vi "tdmsGenToolScaleAllDAQmxTypes.vi"() -> ()   [LabVIEW 2026]
uses:
  <vilib>/Platform/TimedLoop/XDataNode/nitl_modes.ctl
  <vilib>/Platform/TimedLoop/XDataNode/timing_clust.ctl
  <vilib>/Platform/TimedLoop/XDataNode/wakeup.ctl
  <vilib>/DAQmx/read.llb/DAQmx Read (Analog 1D DBL 1Chan NSamp).vi
  <vilib>/DAQmx/create/scale.llb/DAQmx Create Scale (Map Ranges).vi
  <vilib>/DAQmx/create/channels.llb/DAQmx Create Channel (AI-Voltage-Basic).vi
  <vilib>/DAQmx/create/channels.llb/DAQmx Create Channel (AI-Strain-Strain Gage).vi
  <vilib>/DAQmx/create/channels.llb/DAQmx Create Channel (AI-Current-Basic).vi
  <vilib>/DAQmx/create/channels.llb/DAQmx Create Channel (AI-Temperature-RTD).vi
  <vilib>/DAQmx/create/channels.llb/DAQmx Create Channel (AI-Temperature-Thermocouple).vi
  <vilib>/DAQmx/configure/timing.llb/DAQmx Timing (Sample Clock).vi
  <vilib>/DAQmx/configure/task.llb/DAQmx Configure Logging (TDMS).vi
  <vilib>/DAQmx/miscellaneous.llb/DAQmx Fill In Error Info.vi
  <vilib>/platform/TimedLoop/XDataNode/XDataNode.xnode
  <vilib>/Platform/TimedLoop/XDataNode/XDNodeRunTimeDep.lvlib
  <resource>/objmgr/daqmx.rc
panel:
  out "Numeric":i32
  out "Waveform Chart":dbl[](graph)
  in  "DAQType Enum":T1(ring)
  in  "double?":bool
  in  "file format version (2.0)":enum16{"1.0", "2.0"}(ring)=enum."2.0"
  in  "create index file? (T)":bool=TRUE
  in  "byte order (2:little-endian)":T2(ring)
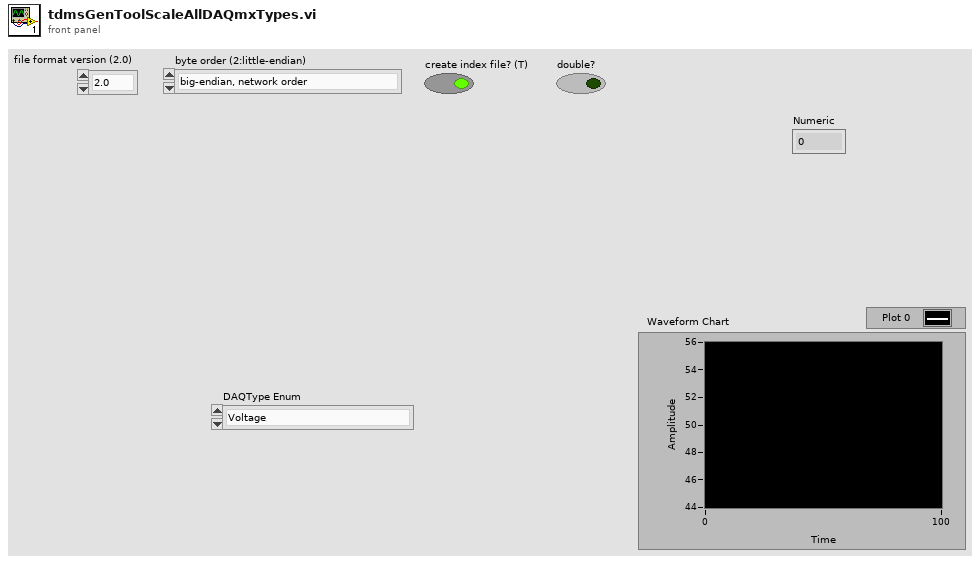
[diagram p1: front panel]
types:
  T1 = enum16{"Voltage", "Current", "RTD", "Thermocouple", "Strain"}
  T2 = enum16{"big-endian, network order", "native, host order", "little-endian"}
  T3 = cluster{"gage factor":dbl, "nominal gage resistance":dbl, "poisson ratio":dbl}
  T4 = typedef "XDNodeRunTimeDep.lvlib/nitl_modes.ctl" = enum32{"No Change", "Process missed periods, maintain original phase", "Discard missed periods, maintain original phase", "Process missed periods, ignore original phase", "Discard missed periods, ignore original phase"}
  T5 = typedef "XDNodeRunTimeDep.lvlib/timing_clust.ctl" = cluster{"Expected End [f-1]":u64, "Actual End [f-1]":u64, "Finished Late? [f-1]":bool, "Expected End [i-1]":u64, "Actual End [i-1]":u64, "Finished Late? [i-1]":bool, "Expected Start [i]":u64, "Actual Start [i]":u64, "Expected Start [f]":u64, "Actual Start [f]":u64, "Source Name":string, "Structure Name":string, "Period":i64, "Deadline":i64, "Offset":i64, "Start":i64, "Priority":i32, "Timeout":i32, "Mode":T4, "Wakeup Reason":T6, "Error":errorcluster, "Source Type":string, "Secondary Source Type":string, "Global End Time":u64, "Global Start Time":u64, "Frame Duration":u64, "Iteration Duration":u64, "Assigned CPU":i32, "I/O Scan Engine Mode":u32}
  T6 = typedef "XDNodeRunTimeDep.lvlib/wakeup.ctl" = enum32{"Normal", "Aborted", "Asynchronous wakeup", "Timing source error", "Timed loop error", "Timeout"}
  T7 = enum16{"open", "open or create", "create or replace", "create", "open (read-only)"}
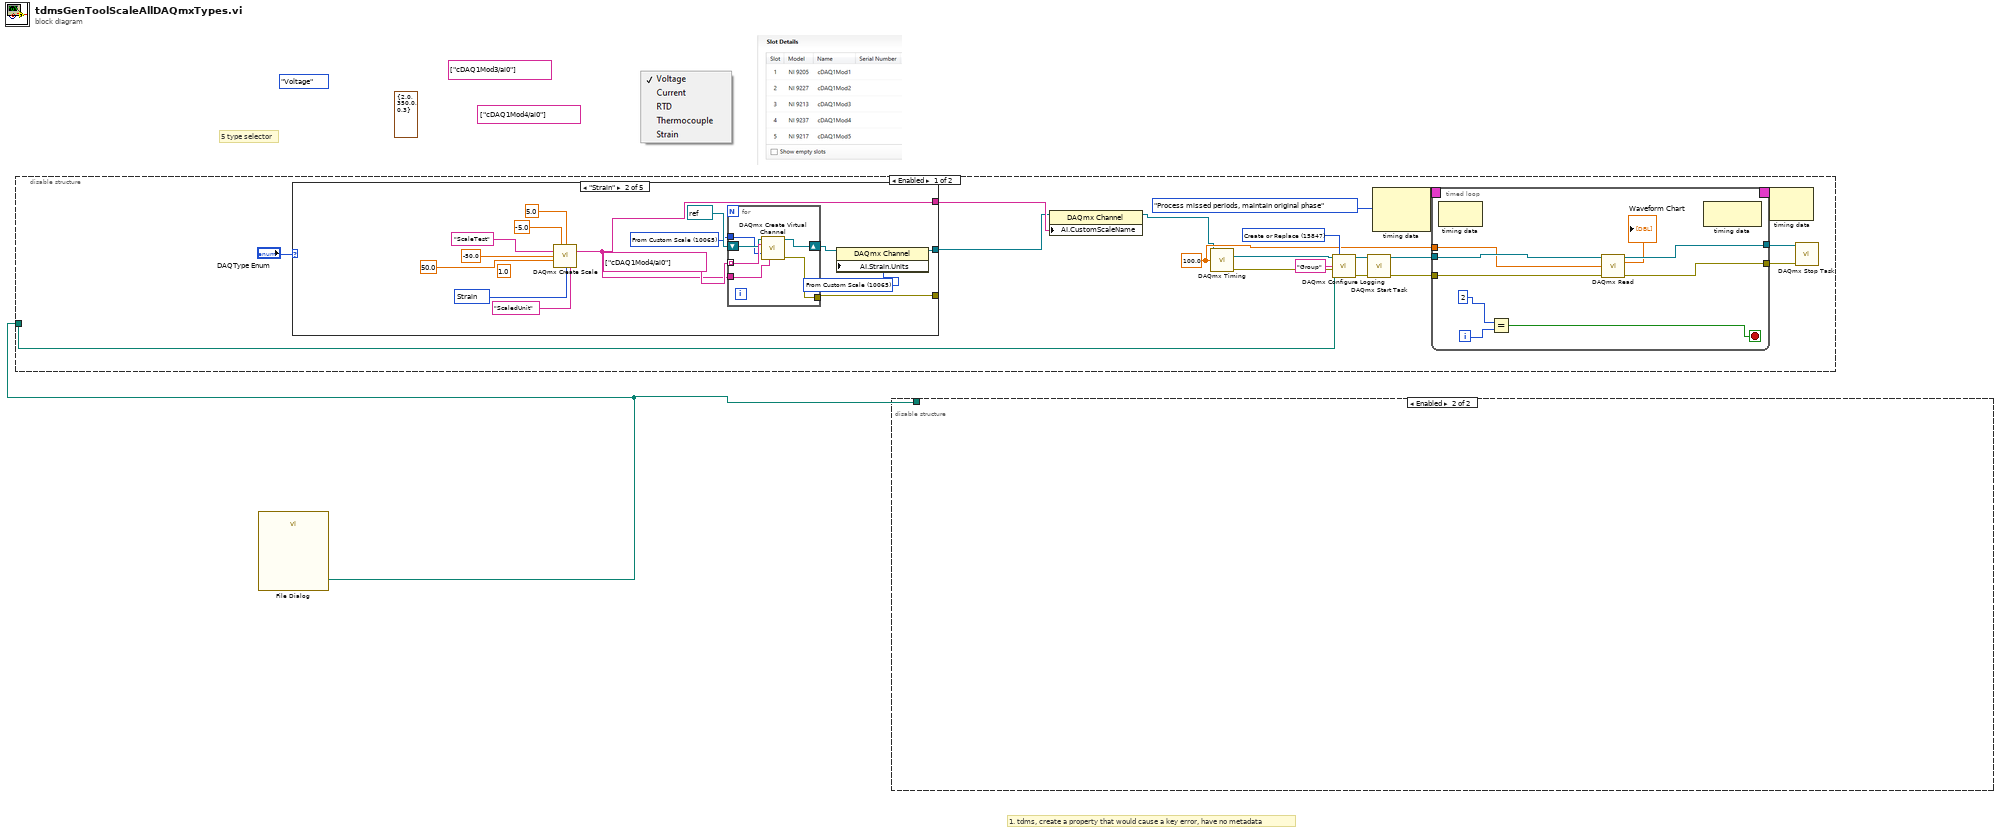
[diagram p0: block diagram]
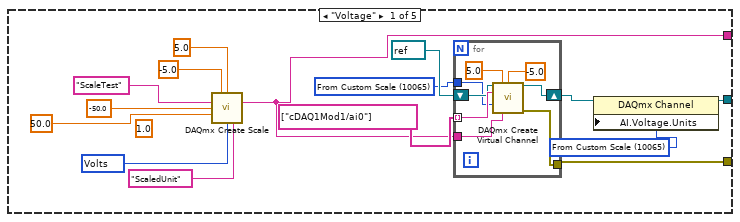
[diagram p2: hidden frame]
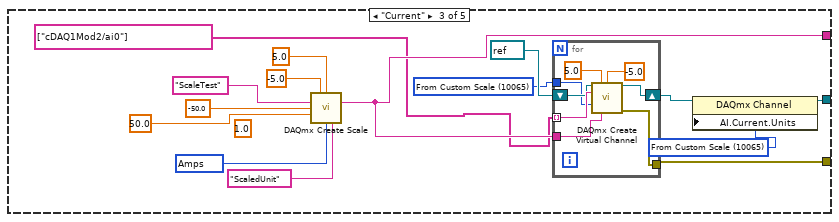
[diagram p3: hidden frame]
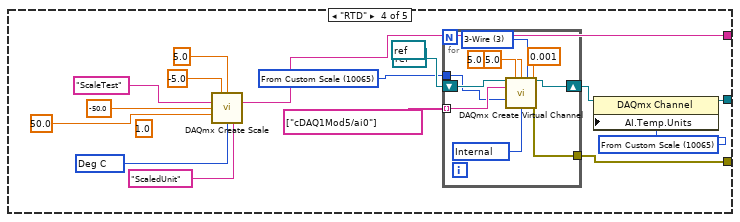
[diagram p4: hidden frame]
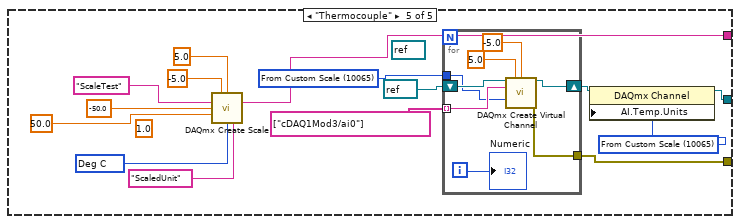
[diagram p5: hidden frame]
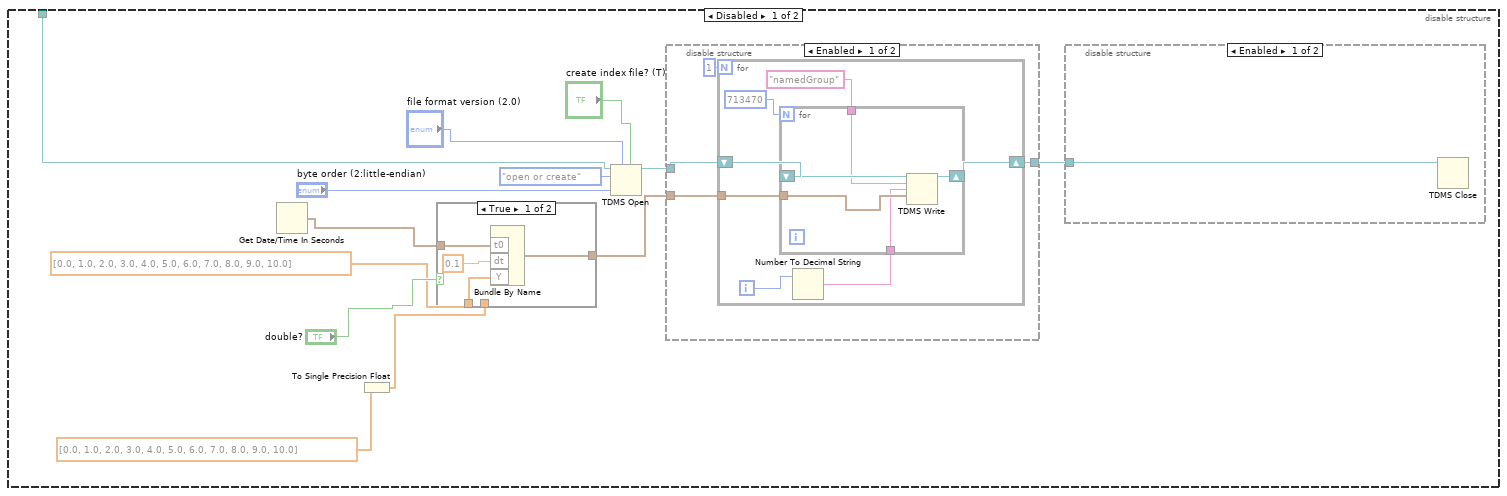
[diagram p7: hidden frame]
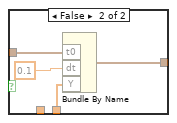
[diagram p10: hidden frame]
diagram:
  (unwired) tag[] ["cDAQ1Mod4/ai0"] ("Voltage Channels")
  (unwired) T3 {"gage factor"=2.0, "nominal gage resistance"=350.0, "poisson ratio"=0.3} ("strain gage information")
  (unwired) tag[] ["cDAQ1Mod3/ai0"] ("Voltage Channels")
  (unwired) T1."Voltage"
  # "5 type selector"
  # "1. tdms, create a property that would cause a key error, have no metadata"
  n1 = call "File Dialog"() -> ("selected path"=w1:path)  [unwired: 12 in, 3 out]
  n2 = disable-structure shown="Enabled" {
    disable-tunnel: w1 -> [w6 _]
    frame Enabled {
      w18 = 15847 items=["Open"=10437, "Open or Create"=15846, "Create or Replace"=15847, "Create"=15848] ("operation")
      w5 = 100.0 ("rate")
      n3 = case shown="\"Strain\"" "DAQType Enum" {
        tunnel: [w30 w53 w75 w102 w127] -> w2
        tunnel: [w35 w58 w79 w88 w113] -> _
        tunnel: [w25 w48 w70 w97 w122] -> w3
        frame "Voltage" {
          (unwired) 1.0 ("y-intercept")
          w29 = 10065 items=["Volts"=10348, "From Custom Scale"=10065, "From TEDS"=12516] ("AI.Voltage.Units")
          w26 = 10348 items=["Volts"=10348, "Amps"=10342, "Watts"=16203, "Deg F"=10144, "Deg C"=10143, "Deg R"=10145, "Kelvins"=10325, "Strain"=10299, "Ohms"=10384, "Hz"=10373, "Seconds"=10364, "Meters"=10219, "Inches"=10379, "Degrees"=10146, "Radians"=10273, "Ticks"=10304, "g"=10186, "m/s^2"=12470, "m/s"=15959, "in/s"=15960, "Pascals"=10081, "Newtons"=15875, "Pounds"=15876, "kgf"=15877, "psi"=15879, "bar"=15880, "Nm"=15881, "oz-in"=15882, "lb-in"=15883, "lb-ft"=15884, "Volts/Volt"=15896, "mVolts/Volt"=15897, "pCoulombs"=16103, "Coulombs"=16102, "From TEDS"=12516] ("pre-scaled units")
          w32 = 10065 items=["Volts"=10348, "From Custom Scale"=10065] ("units")
          n4 = call-poly <vilib>:"DAQmx Create Scale.vi"("pre-scaled minimum"=-5.0, "pre-scaled maximum"=5.0, "name"="ScaleTest", "scaled minimum"=-50.0, "scaled maximum"=50.0, "pre-scaled units"=w26, "scaled units"="ScaledUnit") -> ("scale out"=w25:tag)  [unwired: 7 in, 1 out]
          n5 = for {
            tunnel: [w42] -> w35
            tunnel: tag[] ["cDAQ1Mod1/ai0"] ("Voltage Channels") -> [w41] mode=indexing
            shift-right: [w43] -> w31
            shift-left: refnum<k21> refnum ("task out") -> [w40]
            tunnel: w32 -> [w39]
            tunnel: w25 -> [w38]
            n6 = call-poly <vilib>:"DAQmx Create Virtual Channel.vi"("task in"=w40, "maximum value"=5.0, "minimum value"=-5.0, "physical channels"=w41, "units"=w39, "custom scale name"=w38) -> ("task out"=w43:refnum<k21>, "error out"=w42:errorcluster)  [unwired: 8 in]
          }
          n7 = property class="DAQmx Channel"(reference=w31, "AI.Voltage.Units"=w29) -> (reference out=w30:refnum<k21>)  [unwired: 1 in, 1 out]
        }
        frame "Strain" {
          (unwired) 1.0 ("y-intercept")
          w52 = 10065 items=["Volts"=10348, "From Custom Scale"=10065, "From TEDS"=12516] ("AI.Voltage.Units")
          w49 = 10299 items=["Volts"=10348, "Amps"=10342, "Watts"=16203, "Deg F"=10144, "Deg C"=10143, "Deg R"=10145, "Kelvins"=10325, "Strain"=10299, "Ohms"=10384, "Hz"=10373, "Seconds"=10364, "Meters"=10219, "Inches"=10379, "Degrees"=10146, "Radians"=10273, "Ticks"=10304, "g"=10186, "m/s^2"=12470, "m/s"=15959, "in/s"=15960, "Pascals"=10081, "Newtons"=15875, "Pounds"=15876, "kgf"=15877, "psi"=15879, "bar"=15880, "Nm"=15881, "oz-in"=15882, "lb-in"=15883, "lb-ft"=15884, "Volts/Volt"=15896, "mVolts/Volt"=15897, "pCoulombs"=16103, "Coulombs"=16102, "From TEDS"=12516] ("pre-scaled units")
          w55 = 10065 items=["Volts"=10348, "From Custom Scale"=10065] ("units")
          n8 = call-poly <vilib>:"DAQmx Create Scale.vi"("pre-scaled minimum"=-5.0, "pre-scaled maximum"=5.0, "name"="ScaleTest", "scaled minimum"=-50.0, "scaled maximum"=50.0, "pre-scaled units"=w49, "scaled units"="ScaledUnit") -> ("scale out"=w48:tag)  [unwired: 7 in, 1 out]
          n9 = for {
            tunnel: [w63] -> w58
            tunnel: tag[] ["cDAQ1Mod4/ai0"] ("Voltage Channels") -> [w62] mode=indexing
            shift-right: [w64] -> w54
            shift-left: refnum<k21> refnum ("task out") -> [w61]
            tunnel: w55 -> [w60]
            tunnel: w48 -> [w59]
            n10 = call-poly <vilib>:"DAQmx Create Virtual Channel.vi"("task in"=w61, "physical channels"=w62, "units"=w60, "custom scale name"=w59) -> ("task out"=w64:refnum<k21>, "error out"=w63:errorcluster)  [unwired: 10 in]
          }
          n11 = property class="DAQmx Channel"(reference=w54, "AI.Strain.Units"=w52) -> (reference out=w53:refnum<k21>)  [unwired: 1 in, 1 out]
        }
        frame "Current" {
          (unwired) 1.0 ("y-intercept")
          w74 = 10065 items=["Volts"=10348, "From Custom Scale"=10065, "From TEDS"=12516] ("AI.Voltage.Units")
          w71 = 10342 items=["Volts"=10348, "Amps"=10342, "Watts"=16203, "Deg F"=10144, "Deg C"=10143, "Deg R"=10145, "Kelvins"=10325, "Strain"=10299, "Ohms"=10384, "Hz"=10373, "Seconds"=10364, "Meters"=10219, "Inches"=10379, "Degrees"=10146, "Radians"=10273, "Ticks"=10304, "g"=10186, "m/s^2"=12470, "m/s"=15959, "in/s"=15960, "Pascals"=10081, "Newtons"=15875, "Pounds"=15876, "kgf"=15877, "psi"=15879, "bar"=15880, "Nm"=15881, "oz-in"=15882, "lb-in"=15883, "lb-ft"=15884, "Volts/Volt"=15896, "mVolts/Volt"=15897, "pCoulombs"=16103, "Coulombs"=16102, "From TEDS"=12516] ("pre-scaled units")
          w77 = 10065 items=["Volts"=10348, "From Custom Scale"=10065] ("units")
          n12 = call-poly <vilib>:"DAQmx Create Scale.vi"("pre-scaled minimum"=-5.0, "pre-scaled maximum"=5.0, "name"="ScaleTest", "scaled minimum"=-50.0, "scaled maximum"=50.0, "pre-scaled units"=w71, "scaled units"="ScaledUnit") -> ("scale out"=w70:tag)  [unwired: 7 in, 1 out]
          n13 = for {
            tunnel: [w86] -> w79
            tunnel: tag[] ["cDAQ1Mod2/ai0"] ("Voltage Channels") -> [w85] mode=indexing
            shift-right: [w87] -> w76
            shift-left: refnum<k21> refnum ("task out") -> [w84]
            tunnel: w77 -> [w83]
            tunnel: w70 -> [w82]
            n14 = call-poly <vilib>:"DAQmx Create Virtual Channel.vi"("task in"=w84, "maximum value"=5.0, "minimum value"=-5.0, "physical channels"=w85, "units"=w83, "custom scale name"=w82) -> ("task out"=w87:refnum<k21>, "error out"=w86:errorcluster)  [unwired: 8 in]
          }
          n15 = property class="DAQmx Channel"(reference=w76, "AI.Current.Units"=w74) -> (reference out=w75:refnum<k21>)  [unwired: 1 in, 1 out]
        }
        frame "RTD" {
          (unwired) 1.0 ("y-intercept")
          w101 = 10065 items=["Volts"=10348, "From Custom Scale"=10065, "From TEDS"=12516] ("AI.Voltage.Units")
          w98 = 10143 items=["Volts"=10348, "Amps"=10342, "Watts"=16203, "Deg F"=10144, "Deg C"=10143, "Deg R"=10145, "Kelvins"=10325, "Strain"=10299, "Ohms"=10384, "Hz"=10373, "Seconds"=10364, "Meters"=10219, "Inches"=10379, "Degrees"=10146, "Radians"=10273, "Ticks"=10304, "g"=10186, "m/s^2"=12470, "m/s"=15959, "in/s"=15960, "Pascals"=10081, "Newtons"=15875, "Pounds"=15876, "kgf"=15877, "psi"=15879, "bar"=15880, "Nm"=15881, "oz-in"=15882, "lb-in"=15883, "lb-ft"=15884, "Volts/Volt"=15896, "mVolts/Volt"=15897, "pCoulombs"=16103, "Coulombs"=16102, "From TEDS"=12516] ("pre-scaled units")
          w90 = 10065 items=["Volts"=10348, "From Custom Scale"=10065] ("units")
          (unwired) refnum<k21> refnum ("task out")
          n16 = call-poly <vilib>:"DAQmx Create Scale.vi"("pre-scaled minimum"=-5.0, "pre-scaled maximum"=5.0, "name"="ScaleTest", "scaled minimum"=-50.0, "scaled maximum"=50.0, "pre-scaled units"=w98, "scaled units"="ScaledUnit") -> ("scale out"=w97:tag)  [unwired: 7 in, 1 out]
          n17 = for {
            tunnel: [w111] -> w88
            tunnel: tag[] ["cDAQ1Mod5/ai0"] ("Voltage Channels") -> [w110] mode=indexing
            shift-right: [w112] -> w89
            shift-left: refnum<k21> refnum ("task out") -> [w109]
            tunnel: w90 -> [w105]
            w106 = 3 items=["2-Wire"=2, "3-Wire"=3, "4-Wire"=4] ("resistance configuration")
            w108 = 10200 items=["Internal"=10200, "External"=10167, "None"=10230] ("current excitation source")
            n18 = call-poly <vilib>:"DAQmx Create Virtual Channel.vi"("task in"=w109, "maximum value"=5.0, "minimum value"=-5.0, "resistance configuration"=w106, "physical channels"=w110, "units"=w105, "current excitation value"=0.001, "current excitation source"=w108) -> ("task out"=w112:refnum<k21>, "error out"=w111:errorcluster)  [unwired: 6 in]
          }
          n19 = property class="DAQmx Channel"(reference=w89, "AI.Temp.Units"=w101) -> (reference out=w102:refnum<k21>)  [unwired: 1 in, 1 out]
        }
        frame "Thermocouple" {
          (unwired) 1.0 ("y-intercept")
          w126 = 10065 items=["Volts"=10348, "From Custom Scale"=10065, "From TEDS"=12516] ("AI.Voltage.Units")
          w123 = 10143 items=["Volts"=10348, "Amps"=10342, "Watts"=16203, "Deg F"=10144, "Deg C"=10143, "Deg R"=10145, "Kelvins"=10325, "Strain"=10299, "Ohms"=10384, "Hz"=10373, "Seconds"=10364, "Meters"=10219, "Inches"=10379, "Degrees"=10146, "Radians"=10273, "Ticks"=10304, "g"=10186, "m/s^2"=12470, "m/s"=15959, "in/s"=15960, "Pascals"=10081, "Newtons"=15875, "Pounds"=15876, "kgf"=15877, "psi"=15879, "bar"=15880, "Nm"=15881, "oz-in"=15882, "lb-in"=15883, "lb-ft"=15884, "Volts/Volt"=15896, "mVolts/Volt"=15897, "pCoulombs"=16103, "Coulombs"=16102, "From TEDS"=12516] ("pre-scaled units")
          w115 = 10065 items=["Volts"=10348, "From Custom Scale"=10065] ("units")
          (unwired) refnum<k21> refnum ("task out")
          n20 = call-poly <vilib>:"DAQmx Create Scale.vi"("pre-scaled minimum"=-5.0, "pre-scaled maximum"=5.0, "name"="ScaleTest", "scaled minimum"=-50.0, "scaled maximum"=50.0, "pre-scaled units"=w123, "scaled units"="ScaledUnit") -> ("scale out"=w122:tag)  [unwired: 7 in, 1 out]
          n21 = for {
            tunnel: [w134] -> w113
            tunnel: tag[] ["cDAQ1Mod3/ai0"] ("Voltage Channels") -> [w133] mode=indexing
            shift-right: [w135] -> w114
            shift-left: refnum<k21> refnum ("task out") -> [w132]
            tunnel: w115 -> [w131]
            i -> [w128]
            n22 = call-poly <vilib>:"DAQmx Create Virtual Channel.vi"("task in"=w132, "maximum value"=5.0, "minimum value"=-5.0, "physical channels"=w133, "units"=w131) -> ("task out"=w135:refnum<k21>, "error out"=w134:errorcluster)  [unwired: 9 in]
            "Numeric" <- w128
          }
          n23 = property class="DAQmx Channel"(reference=w114, "AI.Temp.Units"=w126) -> (reference out=w127:refnum<k21>)  [unwired: 1 in, 1 out]
        }
      }
      n24 = property class="DAQmx Channel"(reference=w2, "AI.CustomScaleName"=w3) -> (reference out=w4:refnum<k21>)  [unwired: 1 in, 1 out]
      n25 = call-poly <vilib>:"DAQmx Timing.vi"("task/channels in"=w4, "rate"=w5) -> ("task out"=w16:refnum<k21>, "error out"=w15:errorcluster)  [unwired: 12 in]
      n26 = call-poly <vilib>:"DAQmx Configure Logging.vi"("task/channels in"=w16, "operation"=w18, "file path"=w6, "group name"="Group", "error in"=w15) -> ("task out"=w14:refnum<k21>, "error out"=w13:errorcluster)  [unwired: 9 in]
      n27 = call <vilib>:"DAQmx Start Task.vi"("task/channels in"=w14, "error in"=w13) -> ("task out"=w12:refnum<k21>, "error out"=w11:errorcluster)  [unwired: 12 in]
      n28 = node-c288(nitl_modes."Process missed periods, maintain original phase" ("Mode")) -> (w20:T5)  [unwired: 1 in]
      n29 = timed-loop {
        tunnel: w12 -> [w141]
        tunnel: w11 -> [w140]
        timing: w20 -> [_]
        timing-out: [_] -> w19
        tunnel: [w139] -> w10
        tunnel: [w138] -> w9
        tunnel: w5 -> [w137]
        i -> [w144]
        stop <- w143 stop-if-true
        n30 = node-c288() -> ()  [unwired: 1 in, 1 out]
        n31 = Equal?(x=2, y=w144) -> (x = y?=w143:bool)
        n32 = call-poly <vilib>:"DAQmx Read.vi"("task/channels in"=w141, "number of samples per channel"=w137, "error in"=w140) -> ("task out"=w139:refnum<k21>, "data"=→"Waveform Chart":dbl[], "error out"=w138:errorcluster)  [unwired: 10 in]
        n33 = node-c288() -> ()  [unwired: 1 in, 1 out]
      }
      n34 = node-c288(w19) -> ()  [unwired: 1 out]
      n35 = call <vilib>:"DAQmx Stop Task.vi"("task/channels in"=w10, "error in"=w9) -> ()  [unwired: 12 in, 2 out]
    }
    frame Disabled {
    }
  }
  n36 = disable-structure shown="Enabled" {
    disable-tunnel: w1 -> [w161 _]
    frame Disabled {
      n37 = Get Date/Time In Seconds() -> (seconds since 1Jan1904=w154:timestamp)
      n38 = To Single Precision Float(number=dbl[] [0.0, 1.0, 2.0, 3.0, 4.0, 5.0, 6.0, 7.0, 8.0, 9.0, 10.0] ("Y")) -> (single precision float=w155:sgl[])
      n39 = case shown="True" "double?" {
        tunnel: w154 -> [w185 w189]
        tunnel: [w183 w187] -> w152
        tunnel: dbl[] [0.0, 1.0, 2.0, 3.0, 4.0, 5.0, 6.0, 7.0, 8.0, 9.0, 10.0] ("Y") -> [w182 _]
        tunnel: w155 -> [_ w186]
        frame True {
          n40 = Bundle By Name("t0"=w185, "dt"=0.1, "Y"=w182) -> (w183:waveform(dbl))  [unwired: 1 in]
        }
        frame False {
          n41 = Bundle By Name("t0"=w189, "dt"=0.1, "Y"=w186) -> (w187:waveform(sgl))  [unwired: 1 in]
        }
      }
      n42 = TDMS Open(5:"create index file? (T)", 7:"file format version (2.0)", 9:"byte order (2:little-endian)", 10:T7."open or create" ("operation (0:open)"), 11:w161) -> (3:w163:refnum<k34>)  [unwired: 2 in, 1 out]
      n43 = disable-structure shown="Enabled" {
        disable-tunnel: w163 -> [w167 w180]
        disable-tunnel: [w166 w180] -> w153
        disable-tunnel: w152 -> [w165 _]
        frame Enabled {
          n44 = for {
            N: 1 -> [_]
            tunnel: w165 -> [w170]
            shift-right: [w173] -> w166
            shift-left: w167 -> [w174]
            i -> [w169]
            n45 = Number To Decimal String(number=w169) -> (decimal integer string=w168:string)  [unwired: 1 in]
            n46 = for {
              N: 713470 -> [_]
              shift-right: [w178] -> w173
              shift-left: w174 -> [w179]
              tunnel: "namedGroup" ("group name in (Untitled)") -> [w177]
              tunnel: w170 -> [w176]
              tunnel: w168 -> [w175]
              n47 = TDMS Write(0:w179, 5:w177, 7:w175, 9:w176) -> (4:w178:refnum<k34>)  [unwired: 2 in, 3 out]
            }
          }
        }
        frame Disabled {
        }
      }
      n48 = disable-structure shown="Enabled" {
        disable-tunnel: w153 -> [w181 _]
        frame Enabled {
          n49 = TDMS Close(11:w181) -> ()  [unwired: 1 in, 2 out]
        }
        frame Disabled {
        }
      }
    }
    frame Enabled {
    }
  }
